vi "Main.vi"() -> ()   [LabVIEW 2017]
uses:
  SSR_class/SSR.lvclass
panel:
  in  "SSR Status to Set":bool
  in  "SSR Channel Number (Zero Based)":i32
  out "DO Status":bool[](array[boolean])
  in  "Quit Program":bool
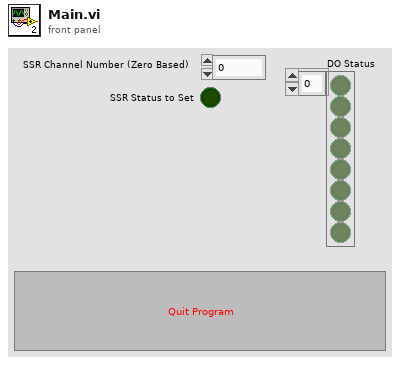
[diagram p1: front panel]
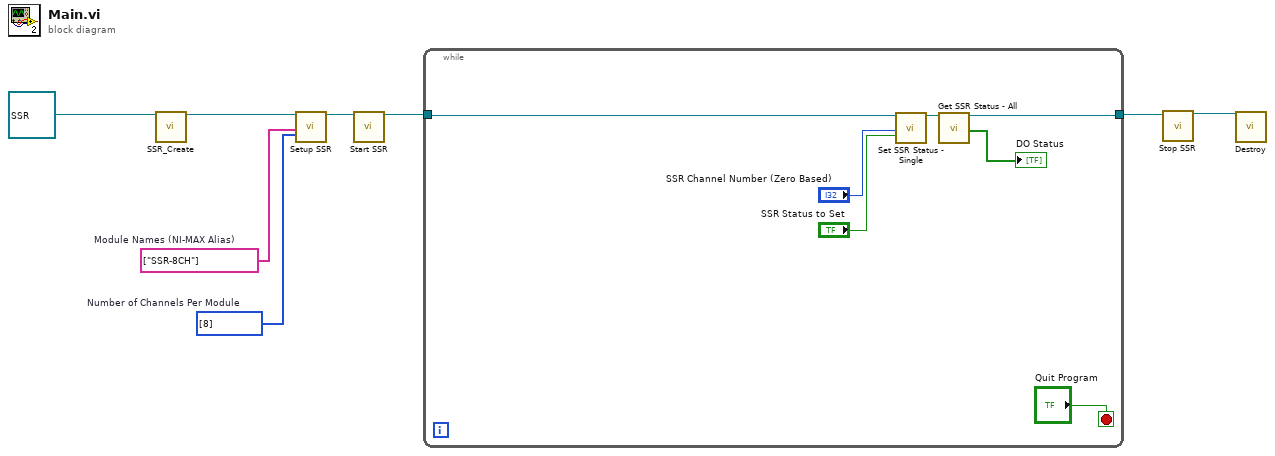
[diagram p0: block diagram]
diagram:
  w1 = u32[] [8]  # Number of Channels Per Module
  w2 = string[] ["SSR-8CH"]  # Module Names (NI-MAX Alias)
  n1 = call "SSR_Create.vi"("reference in"=refnum<class "SSR.lvclass"> refnum ("SSR")) -> ("reference out"=w7:refnum<class "SSR.lvclass">)  [unwired: 17 in, 1 out]
  n2 = call-dynamic "Setup SSR.vi"("reference in"=w7, "Module Names (NI-MAX Alias)"=w2, "Number of Channels Per Module"=w1) -> ("reference out"=w6:refnum<class "SSR.lvclass">)  [unwired: 15 in, 1 out]
  n3 = call-dynamic "Start SSR.vi"("reference in"=w6) -> ("reference out"=w5:refnum<class "SSR.lvclass">)  [unwired: 17 in, 1 out]
  n4 = while {
    tunnel: w5 -> [w9]
    tunnel: [w14] -> w4
    stop <- "Quit Program" stop-if-true
    n5 = call-dynamic "Set SSR Status - Single.vi"("reference in"=w9, "SSR Channel Number (Zero Based)"="SSR Channel Number (Zero Based)", "SSR Status to Set"="SSR Status to Set") -> ("reference out"=w10:refnum<class "SSR.lvclass">)  [unwired: 14 in, 2 out]
    n6 = call-dynamic "Get SSR Status - All.vi"("reference in"=w10) -> ("reference out"=w14:refnum<class "SSR.lvclass">, "All DO Status"=→"DO Status":bool[])  [unwired: 16 in, 1 out]
  }
  n7 = call-dynamic "Stop SSR.vi"("reference in"=w4) -> ("reference out"=w3:refnum<class "SSR.lvclass">)  [unwired: 17 in, 1 out]
  n8 = call-dynamic "Destroy.vi"("reference in"=w3) -> ()  [unwired: 17 in, 2 out]
